vi "ValidPosition(SubVI).vi"(1 "detection":bool, 2 "BUff":dbl[](array[numeric]), 3 "Postion":dbl[](array[numeric])) -> (0 "Valid Position":dbl[](array[numeric]))   [LabVIEW 2017]
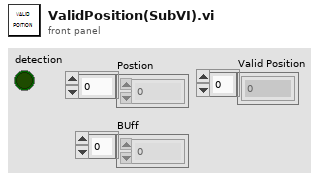
[diagram p1: front panel]
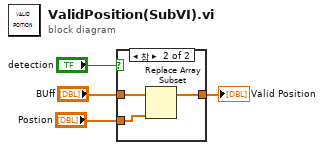
[diagram p0: block diagram]
diagram:
  n1 = case shown="참" "detection" {
    tunnel: "BUff" -> [w5 w8]
    tunnel: "Postion" -> [_ w7]
    tunnel: [w5 w6] -> w1
    frame False {
    }
    frame True {
      n2 = Replace Array Subset(array=w8, new element=w7) -> (w6:dbl[])  [unwired: 1 in]
    }
  }
  "Valid Position" <- w1
